vi "Focus Move Relative.vi"(8 "error in (no error)":errorcluster, 9 "Counts":i32, 10 "Motor (0:n-1)":i32, 11 "ArduinoFocus in":refnum<class "ArduinoFocus.lvclass">) -> (0 "error out":errorcluster, 2 "response":string, 3 "ArduinoFocus out":refnum<class "ArduinoFocus.lvclass">)   [LabVIEW 2022 SP3, in "ArduinoFocus.lvclass"]
uses:
  ArduinoFocus.lvclass
  ArduinoFocus.lvclass/ArduinoFocus.ctl
  Filter Wheel/Filter Wheel Arduino Control/FW Arduino Control.lvclass
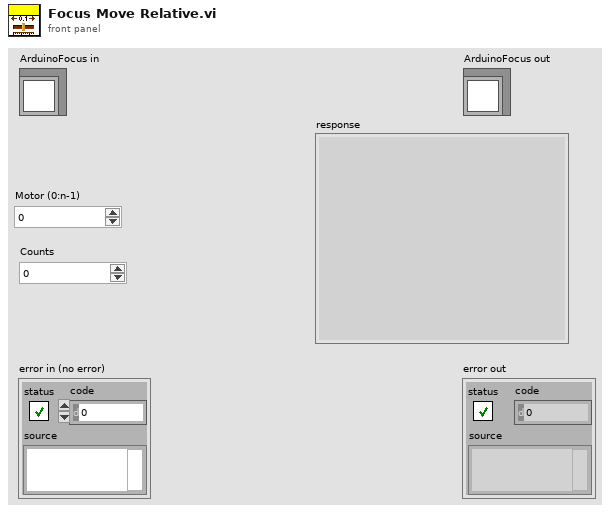
[diagram p1: front panel]
types:
  T1 = typedef "arduino Motor Control cluster Command.ctl" = cluster{"Direction":bool, "NUMBER OF  STEPS":u32, "SPEED STEPS/SEC":u16, "ACC/DECEL STEPS/SEC^2":u16, "EN/DIS?":bool}
  T2 = typedef "ArduinoFocus.lvclass/Arduino Focus cluster Settings.ctl" = cluster{"Port":refnum<visa-resource-name>, "Homing Parameters":T1, "Positions":i32[], "Homed":bool[]}
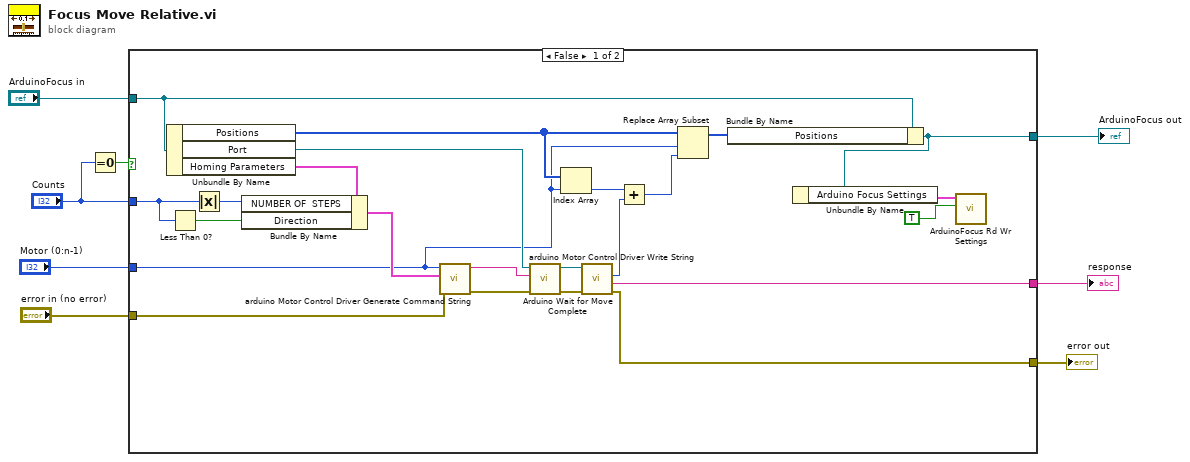
[diagram p0: block diagram]
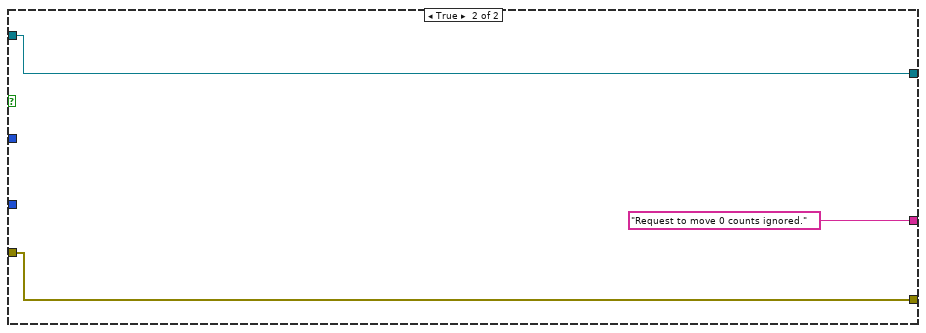
[diagram p2: hidden frame]
diagram:
  n1 = Equal To 0?(x="Counts") -> (x = 0?=w1:bool)
  n2 = case shown="False" w1 {
    tunnel: "Counts" -> [w25 _]
    tunnel: "error in (no error)" -> [w22 w33]
    tunnel: "Motor (0:n-1)" -> [w16 _]
    tunnel: [w15 w33] -> w6
    tunnel: "ArduinoFocus in" -> [w14 w34]
    tunnel: [w11 w34] -> w4
    tunnel: [w12 "Request to move 0 counts ignored." ("response")] -> w3
    frame False {
      n3 = Unbundle By Name(w14) -> ("Positions"=w18:i32[], "Port"=w21:refnum<visa-resource-name>, "Homing Parameters"=w27:T1)
      n4 = Less Than 0?(x=w25) -> (x < 0?=w24:bool)
      n5 = Absolute Value(x=w25) -> (abs(x)=w26:i32)
      n6 = Bundle By Name(cluster=w27, "NUMBER OF  STEPS"=w26, "Direction"=w24) -> (w23:T1)
      n7 = call "arduino Motor Control Driver Generate Command String.vi"("error in (no error)"=w22, "Command"=w23, "MOTOR NUMBER"=w16) -> ("error out"=w30:errorcluster, "Cmd String"=w31:string)  [unwired: 7 in]
      n8 = call "arduino Motor Control Driver Write String.vi"("error in (no error)"=w30, "String"=w31, "VISA resource name"=w21) -> ("error out"=w28:errorcluster, "VISA resource name out"=w29:refnum<visa-resource-name>)  [unwired: 7 in]
      n9 = Index Array(array=w18, index=w16) -> (element=w20:i32)
      n10 = call "Arduino Wait for Move Complete.vi"("error in (no error)"=w28, "reference"=w29) -> ("error out"=w15:errorcluster, "response"=w12:string, "distance"=w19:i32)  [unwired: 6 in, 1 out]
      n11 = Add(x=w20, y=w19) -> (x+y=w17:i32)
      n12 = Replace Array Subset(array=w18, new element=w17, index=w16) -> (w13:i32[])
      n13 = Bundle By Name(cluster=w14, "Positions"=w13) -> (w11:refnum<class "ArduinoFocus.lvclass">)
      n14 = Unbundle By Name(w11) -> ("Arduino Focus Settings"=w10:T2)
      n15 = call "ArduinoFocus Rd Wr Settings.vi"("Write? (F:Read)"=TRUE, "Arduino Focus Settings"=w10) -> ()  [unwired: 8 in, 2 out]
    }
    frame True {
    }
  }
  "error out" <- w6
  "ArduinoFocus out" <- w4
  "response" <- w3
